vi "read_attributes.vi"(8 "error in (no error)":errorcluster, 11 "LassoLars in":refnum<class "LassoLars.lvclass">) -> (0 "error out":errorcluster, 2 "attributes":T1, 3 "LassoLars out":refnum<class "LassoLars.lvclass">)   [LabVIEW 2020, in "LassoLars.lvclass"]
uses:
  LassoLars.lvclass
  Controls/lasso_lars_attributes.ctl
  LassoLars.lvclass/LassoLars.ctl
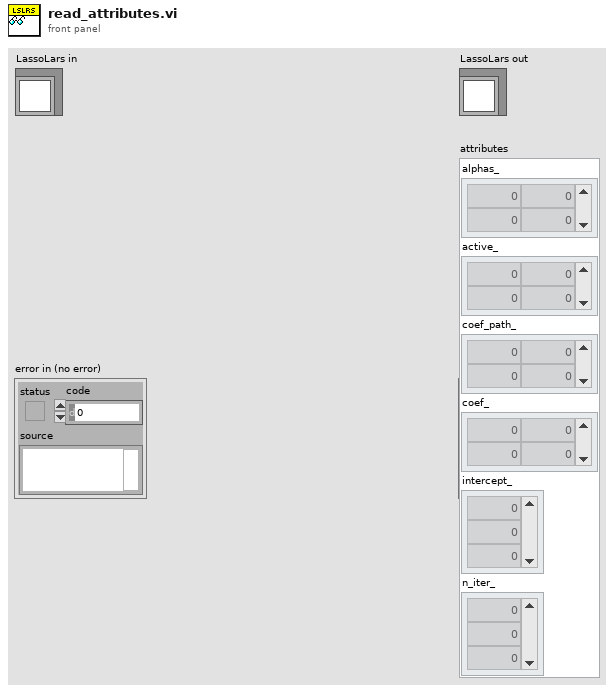
[diagram p1: front panel]
types:
  T1 = typedef "lasso_lars_attributes.ctl" = cluster{"alphas_":dbl[][], "active_":dbl[][], "coef_path_":dbl[][][], "coef_":dbl[][], "intercept_":dbl[], "n_iter_":dbl[]}
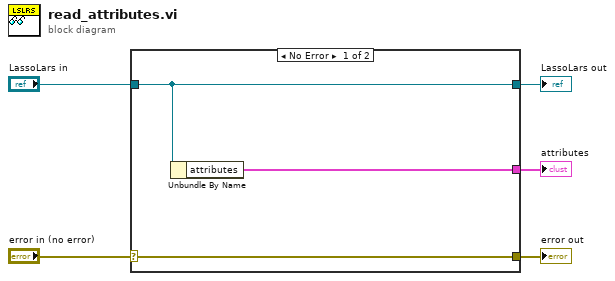
[diagram p0: block diagram]
diagram:
  n1 = case shown="No Error" "error in (no error)" {
    selector: "error in (no error)" -> [w8 w9]
    tunnel: [w8 w9] -> w4
    tunnel: [w7 w10] -> w2
    tunnel: "LassoLars in" -> [w7 w10]
    tunnel: [w6 _] -> w1
    frame No Error {
      n2 = Unbundle By Name(w7) -> ("attributes"=w6:T1)
    }
    frame Error {
    }
  }
  "error out" <- w4
  "LassoLars out" <- w2
  "attributes" <- w1
